vi "MFLI -- publish -- get freq.vi"(7 "publisher action":T1, 9 "Voltage IN (V)":cdb=1.133070214302279+0.0i, 10 "freq IN (Hz)":dbl=1.133070214302279) -> (1 "Voltage out (V)":cdb=1.133070214302279+0.0i, 2 "freq out (Hz)":dbl=1.133070214302279)   [LabVIEW 2017]
uses:
  publisher action.ctl
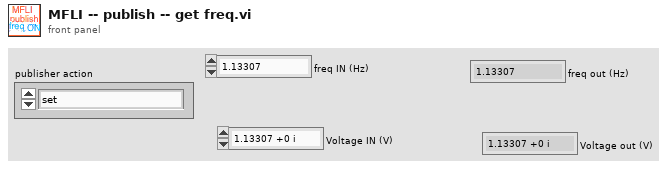
[diagram p1: front panel]
types:
  T1 = typedef "publisher action.ctl" = enum16{"set", "get"}
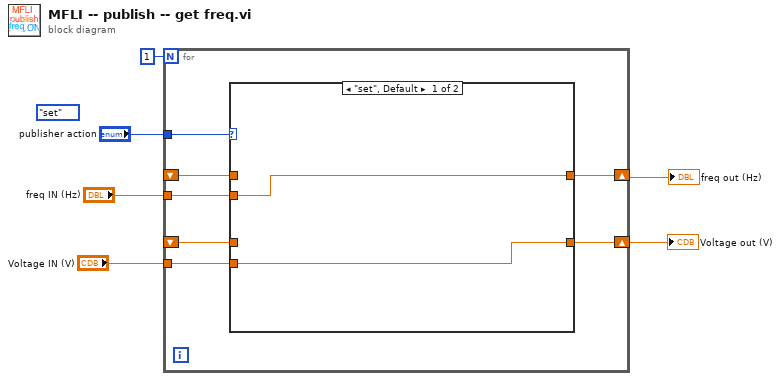
[diagram p0: block diagram]
diagram:
  (unwired) publisher_action."set" ("publisher action")
  n1 = for {
    N: 1 -> [_]
    tunnel: "publisher action" -> [w13]
    tunnel: "freq IN (Hz)" -> [w11]
    shift-right: [w12] -> w2
    shift-left: _ -> [w10]
    shift-right: [w9] -> w1
    shift-left: _ -> [w7]
    tunnel: "Voltage IN (V)" -> [w8]
    n2 = case shown="\"set\", Default" w13 {
      tunnel: [w15 w17] -> w12
      tunnel: w11 -> [w15 _]
      tunnel: w10 -> [_ w17]
      tunnel: [w14 w16] -> w9
      tunnel: w8 -> [w14 _]
      tunnel: w7 -> [_ w16]
      frame "set", Default {
      }
      frame "get" {
      }
    }
  }
  "Voltage out (V)" <- w1
  "freq out (Hz)" <- w2
